vi "Interpolate 2D Scattered_Barycentric.vi"(0 "X In":dbl[](array[numeric]), 5 "Y In":dbl[](array[numeric]), 7 "x":dbl, 9 "y":dbl, 11 "area in":dbl) -> (4 "X Out":dbl[](array[numeric]), 6 "Y Out":dbl[](array[numeric]), 10 "W":dbl[](array[numeric]), 15 "area out":dbl)   [LabVIEW 2017, in "NI_AAL_Interpolation.lvlib"]
uses:
  <vilib>/gmath/NI_AAL_Interpolation.lvlib
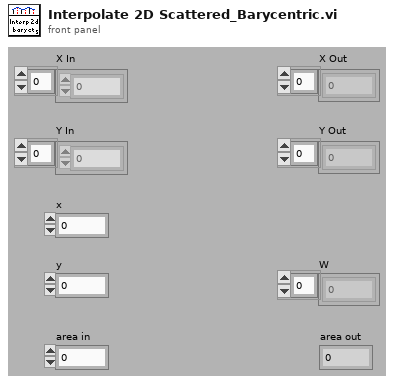
[diagram p1: front panel]
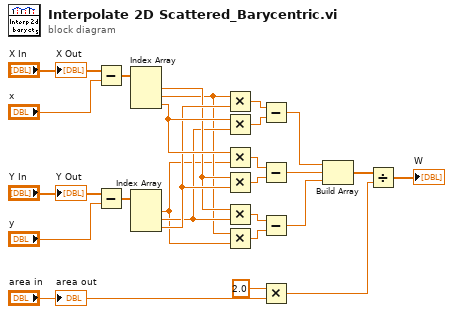
[diagram p0: block diagram]
diagram:
  n1 = Subtract(x="X In", y="x") -> (x-y=w26:dbl[])
  n2 = Subtract(x="Y In", y="y") -> (x-y=w24:dbl[])
  n3 = Index Array(array=w26) -> (element #1=w20:dbl, element #2=w18:dbl, element #3=w22:dbl)  [unwired: 3 in]
  n4 = Index Array(array=w24) -> (element #1=w17:dbl, element #2=w19:dbl, element #3=w21:dbl)  [unwired: 3 in]
  n5 = Multiply(x=w18, y=w21) -> (x*y=w16:dbl)
  n6 = Multiply(x=w22, y=w19) -> (x*y=w15:dbl)
  n7 = Multiply(x=w22, y=w17) -> (x*y=w11:dbl)
  n8 = Multiply(x=w20, y=w21) -> (x*y=w14:dbl)
  n9 = Multiply(x=w20, y=w19) -> (x*y=w13:dbl)
  n10 = Multiply(x=w18, y=w17) -> (x*y=w12:dbl)
  n11 = Subtract(x=w16, y=w15) -> (x-y=w9:dbl)
  n12 = Subtract(x=w11, y=w14) -> (x-y=w10:dbl)
  n13 = Subtract(x=w13, y=w12) -> (x-y=w8:dbl)
  n14 = Multiply(x=2.0, y="area in") -> (x*y=w5:dbl)
  n15 = Build Array(w9, w10, w8) -> (w6:dbl[])
  n16 = Divide(x=w6, y=w5) -> (x/y=→"W":dbl[])
  "X Out" <- "X In"
  "Y Out" <- "Y In"
  "area out" <- "area in"
